vi "Write PWM Outputs.vi"(0 "FPGE Ref":T1, 1 "Frequency":i32, 2 "Controller CMDs IN":dbl[](array[numeric]), 3 "Stagger Counter":i32, 4 "Stagger Time (ms)":i32, 5 "Run Profile":bool) -> (14 "Controller CMDs OUT":dbl[](array[numeric]))   [LabVIEW 2013]
uses:
  Controls/FPGA_Reference.ctl
  <vilib>/Utility/error.llb/Error Cluster From Error Code.vi
  <vilib>/rvi/errors/niLvFpgaAdjustHostInterfaceError.vi
  <vilib>/rvi/interface/nirviReadWriteControl/nirviReadWriteControl.xnode
  FPGA/bitfiles/TI sbRIO PWM (FPGA) v1.0.lvbitx
  NiFpgaLv.dll
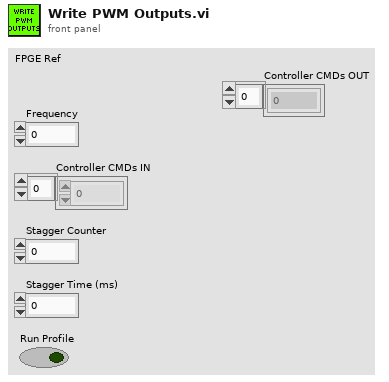
[diagram p1: front panel]
types:
  T1 = typedef "FPGA_Reference.ctl" = refnum<k20>
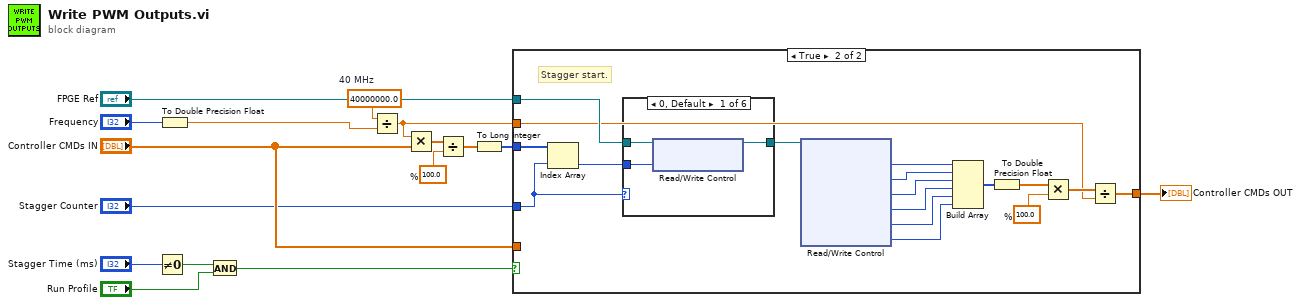
[diagram p0: block diagram]
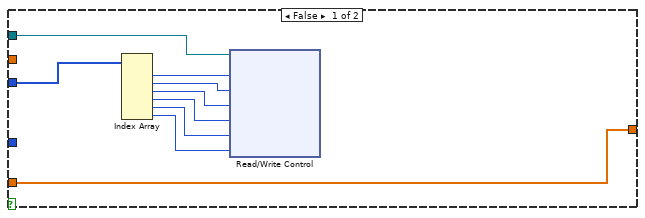
[diagram p2: hidden frame]
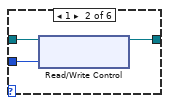
[diagram p3: hidden frame]
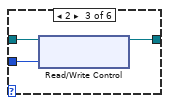
[diagram p4: hidden frame]
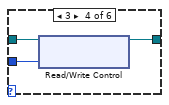
[diagram p5: hidden frame]
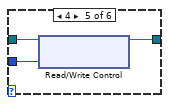
[diagram p6: hidden frame]
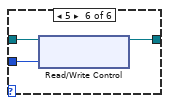
[diagram p7: hidden frame]
diagram:
  w8 = 40000000.0  # 40 MHz
  w10 = 100.0  # %
  n1 = Not Equal To 0?(x="Stagger Time (ms)") -> (x != 0?=w3:bool)
  n2 = To Double Precision Float(number="Frequency") -> (double precision float=w5:dbl)
  n3 = And(x=w3, y="Run Profile") -> (x .and. y?=w1:bool)
  n4 = Divide(x=w8, y=w5) -> (x/y=w14:dbl)
  n5 = Multiply(x=w14, y="Controller CMDs IN") -> (x*y=w11:dbl[])
  n6 = Divide(x=w11, y=w10) -> (x/y=w9:dbl[])
  n7 = To Long Integer(number=w9) -> (32bit integer=w7:i32[])
  n8 = case shown="True" w1 {
    tunnel: w7 -> [w25 w42]
    tunnel: "FPGE Ref" -> [w17 w41]
    tunnel: "Stagger Counter" -> [_ w39]
    tunnel: w14 -> [_ w27]
    tunnel: [w24 w26] -> w15
    tunnel: "Controller CMDs IN" -> [w24 _]
    frame False {
      n9 = Index Array(array=w25) -> (element #1=w23:i32, element #2=w22:i32, element #3=w21:i32, element #4=w20:i32, element #5=w19:i32, element #6=w18:i32)  [unwired: 6 in]
      n10 = xnode "Read/Write Control"("FPGA VI Reference In"=w17, "Duty (Ticks) 1"=w23, "Duty (Ticks) 2"=w22, "Duty (Ticks) 3"=w21, "Duty (Ticks) 4"=w20, "Duty (Ticks) 5"=w19, "Duty (Ticks) 6"=w18) -> ()  [unwired: 1 in, 2 out]
    }
    frame True {
      w29 = 100.0  # %
      # "Stagger start."
      n11 = Index Array(array=w42, index=w39) -> (element=w40:i32)
      n12 = case shown="0, Default" w39 {
        tunnel: w41 -> [w45 w48 w51 w54 w57 w60]
        tunnel: w40 -> [w44 w47 w50 w53 w56 w59]
        tunnel: [w43 w46 w49 w52 w55 w58] -> w38
        frame 0, Default {
          n13 = xnode "Read/Write Control"("FPGA VI Reference In"=w45, "Duty (Ticks) 1"=w44) -> ("FPGA VI Reference Out"=w43:T1)  [unwired: 1 in, 1 out]
        }
        frame 1 {
          n14 = xnode "Read/Write Control"("FPGA VI Reference In"=w48, "Duty (Ticks) 2"=w47) -> ("FPGA VI Reference Out"=w46:T1)  [unwired: 1 in, 1 out]
        }
        frame 2 {
          n15 = xnode "Read/Write Control"("FPGA VI Reference In"=w51, "Duty (Ticks) 3"=w50) -> ("FPGA VI Reference Out"=w49:T1)  [unwired: 1 in, 1 out]
        }
        frame 3 {
          n16 = xnode "Read/Write Control"("FPGA VI Reference In"=w54, "Duty (Ticks) 4"=w53) -> ("FPGA VI Reference Out"=w52:T1)  [unwired: 1 in, 1 out]
        }
        frame 4 {
          n17 = xnode "Read/Write Control"("FPGA VI Reference In"=w57, "Duty (Ticks) 5"=w56) -> ("FPGA VI Reference Out"=w55:T1)  [unwired: 1 in, 1 out]
        }
        frame 5 {
          n18 = xnode "Read/Write Control"("FPGA VI Reference In"=w60, "Duty (Ticks) 6"=w59) -> ("FPGA VI Reference Out"=w58:T1)  [unwired: 1 in, 1 out]
        }
      }
      n19 = xnode "Read/Write Control"("FPGA VI Reference In"=w38) -> ("Duty (Ticks) 1"=w37:i32, "Duty (Ticks) 2"=w36:i32, "Duty (Ticks) 3"=w35:i32, "Duty (Ticks) 4"=w34:i32, "Duty (Ticks) 5"=w33:i32, "Duty (Ticks) 6"=w32:i32)  [unwired: 1 in, 2 out]
      n20 = Build Array(w37, w36, w35, w34, w33, w32) -> (w31:i32[])
      n21 = To Double Precision Float(number=w31) -> (double precision float=w30:dbl[])
      n22 = Multiply(x=w30, y=w29) -> (x*y=w28:dbl[])
      n23 = Divide(x=w28, y=w27) -> (x/y=w26:dbl[])
    }
  }
  "Controller CMDs OUT" <- w15
